vi "Send Stream Command.vi"(7 "Data":string, 8 "error in (no error)":errorcluster, 9 "Command":string, 10 "Device Number":string, 11 "VISA resource name":refnum<visa-resource-name>) -> (0 "error out":errorcluster, 3 "VISA resource name out":refnum<visa-resource-name>)   [LabVIEW 2013, in "Zaber A Series.lvlib"]
doc: "Sends a command to the device and handles the AGAIN responses that can happen with streamed commands. Devices that support live streaming can queue up a number of commands for sequential execution, but when the queue is full the device will respond to new commands with AGAIN until some commands complete and free up space in the queue. This VI will block until the device either accepts the new command or produces an error.\n\nThis VI requires that the Initialize VI has been called with the same serial port."
uses:
  Zaber A Series.lvlib
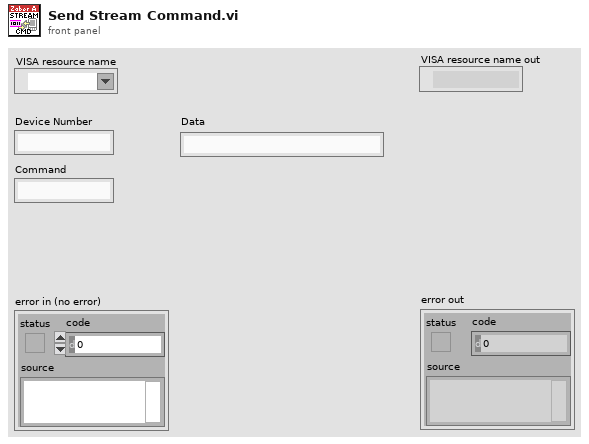
[diagram p1: front panel]
types:
  T1 = cluster{"Device":string, "Axis":string, "Reply Flag":string, "Status":string, "Warning Flags":string, "Data":string}[]
  T2 = cluster{"Device":string, "Axis":string, "Reply Flag":string, "Status":string, "Warning Flags":string, "Data":string}
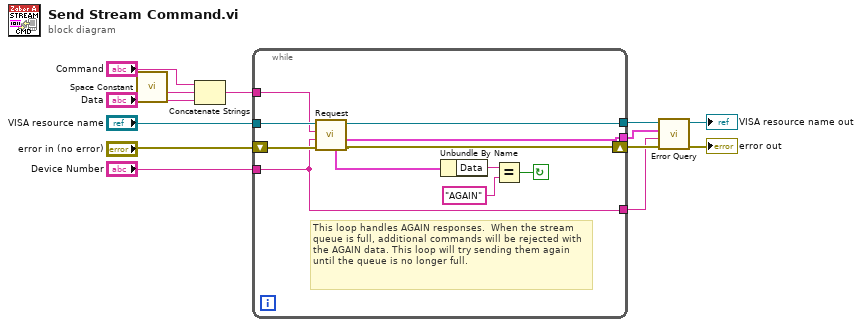
[diagram p0: block diagram]
diagram:
  n1 = call <vilib>:"Space Constant.vi"() -> ("String"=w7:string)
  n2 = Concatenate Strings("Command", w7, "Data") -> (w4:string)
  n3 = while {
    tunnel: [w20] -> w11
    tunnel: "Device Number" -> [w15]
    tunnel: "VISA resource name" -> [w21]
    tunnel: w4 -> [w19]
    tunnel: [w16] -> w3
    tunnel: [w15] -> w1
    shift-right: [w17] -> w9
    shift-left: "error in (no error)" -> [w18]
    stop <- w22 continue-if-true
    # "This loop handles AGAIN responses.  When the stream queue is full, additional commands will be rejected with the AGAIN data. This loop will try sending them again until the queue is no longer full."
    n4 = call "Request.vi"("error in (no error)"=w18, "Device and Axis"=w15, "Command String"=w19, "VISA resource name"=w21) -> ("error out"=w17:errorcluster, "Response Bundle Array"=w16:T1, "VISA resource name out"=w20:refnum<visa-resource-name>, "First Response Bundle"=w14:T2)  [unwired: 2 in, 2 out]
    n5 = Unbundle By Name(w14) -> ("Data"=w23:string)
    n6 = Equal?(x=w23, y="AGAIN") -> (x = y?=w22:bool)
  }
  n7 = call "Error Query.vi"("error in (no error)"=w9, "Device and Axis"=w1, "Previous Response Bundle Array"=w3, "VISA resource name"=w11) -> ("error out"=→"error out":errorcluster, "VISA resource name out"=→"VISA resource name out":refnum<visa-resource-name>)  [unwired: 4 in, 2 out]
